vi "fitting modified.vi"(0 "fitting type":i8(ring), 5 "2D data":dbl[][](array[numeric]), 9 "force guess?":bool, 11 "intial guess value":dbl[](array[numeric])) -> (3 "number of function calls":i32 caption="function calling times", 6 "best fit":dbl[][](array[numeric]), 10 "best fit parameters":dbl[](array[numeric]), 15 "error out":errorcluster)   [LabVIEW 2015]
uses:
  <vilib>/gmath/NumericalOptimization/Nonlinear Curve Fit LM.vi
  Abort.vi
  <vilib>/gmath/NI_Gmath.lvlib
panel:
  out "Abort":bool
  in  "stop":bool
  out "Array 2":dbl[][](array[numeric])
  out "Array":i32[](array[numeric])
  out "output array":dbl[](array[numeric])
  out "size(s) 4":i32[](array[numeric])
  out "size(s) 3":i32[](array[numeric])
  out "size(s) 2":i32[](array[numeric])
  out "size(s)":i32[](array[numeric])
  out "initial value 3":dbl[](array[numeric])
  out "sub3":dbl[][](array[numeric])
  out "split 2":dbl
  out "split 1":dbl
  in  "initial value 2":dbl[](array[numeric])
  in  "initial value 1":dbl[](array[numeric])
  in  "sub2":dbl[][](array[numeric])
  in  "sub1":dbl[][](array[numeric])
  in  "yc":dbl[](array[numeric])
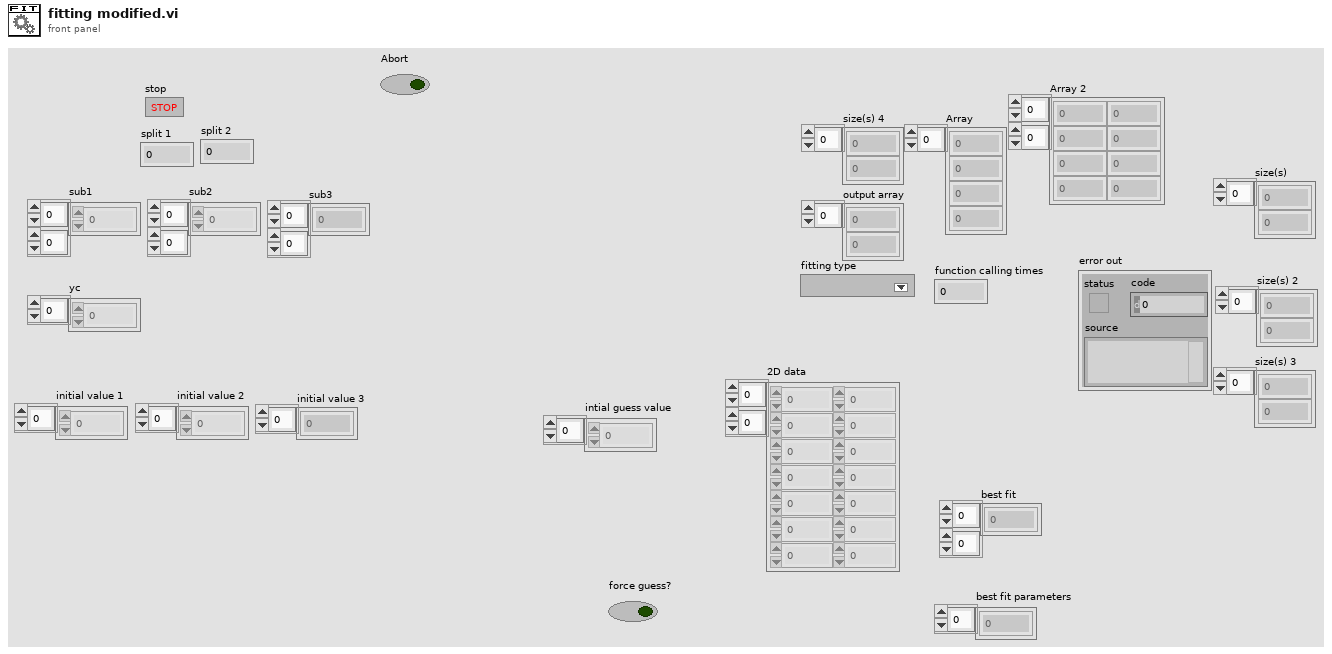
[diagram p1: front panel]
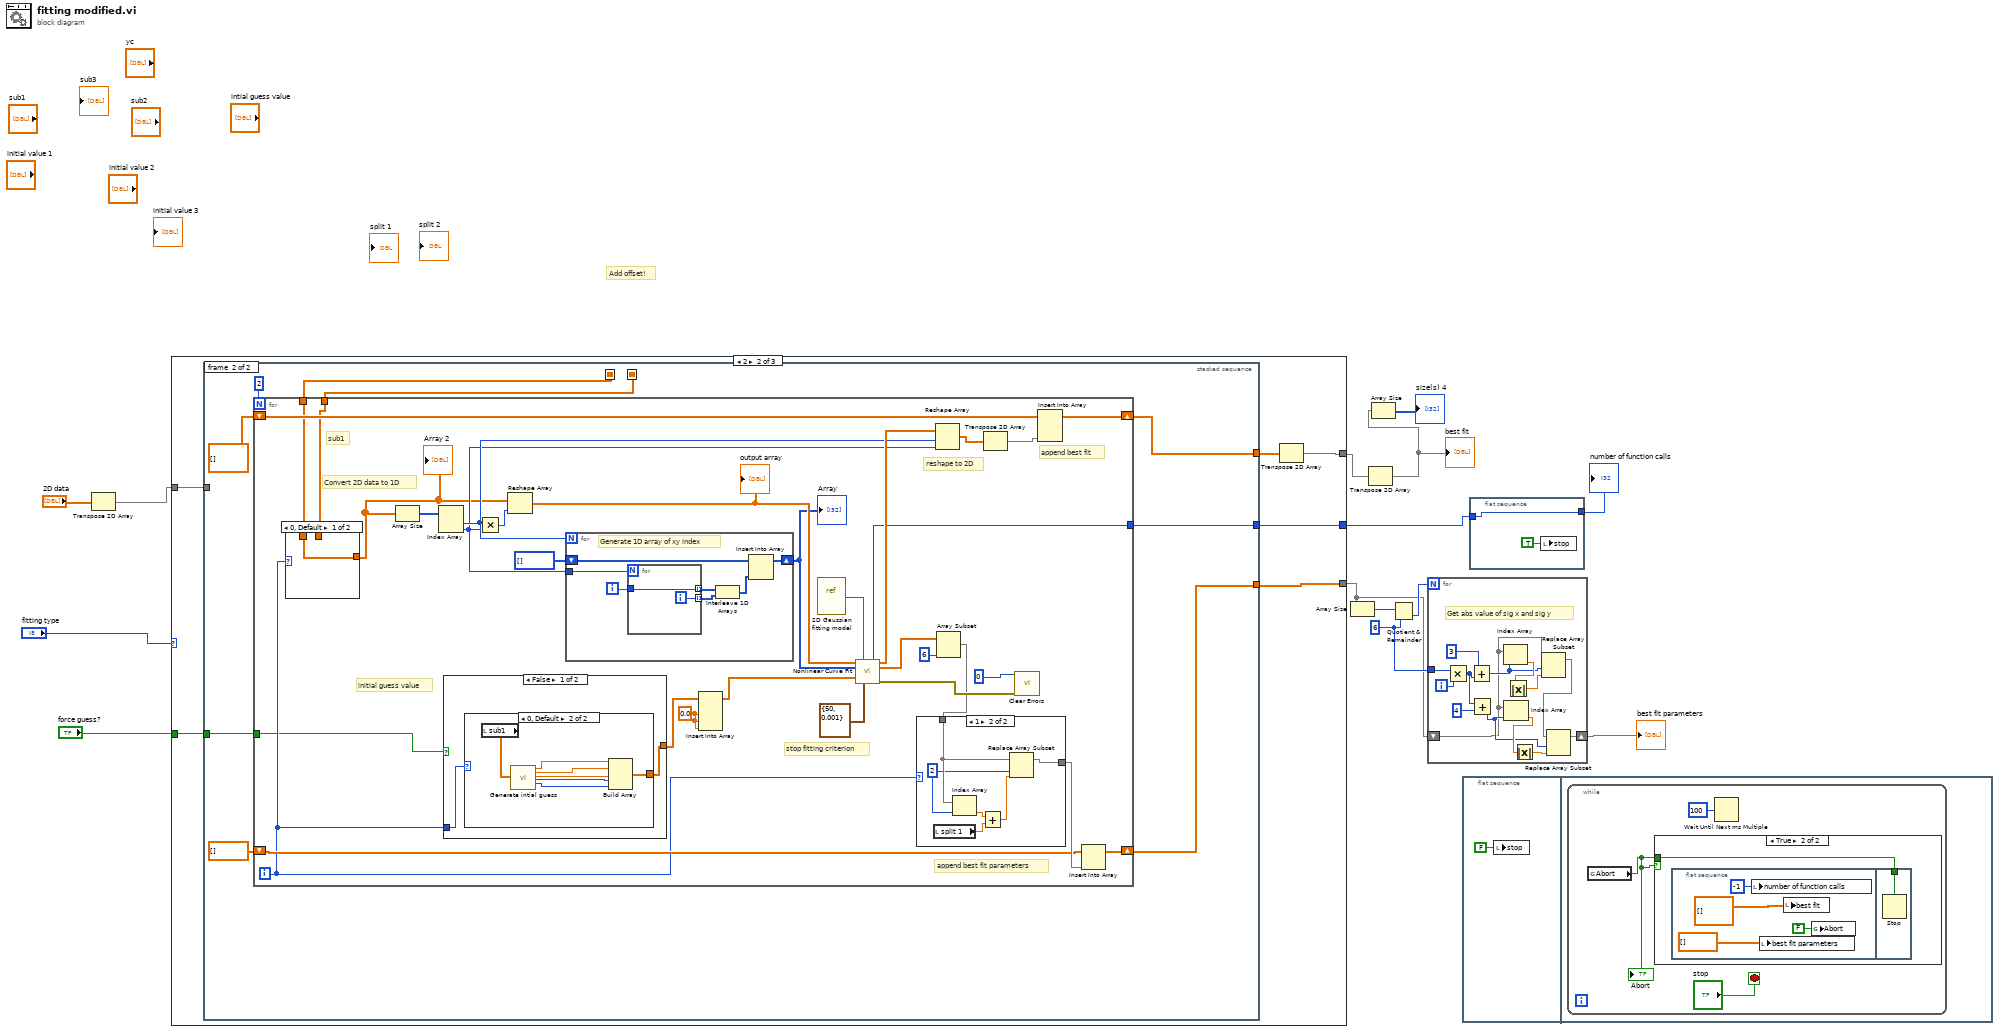
[diagram p0: block diagram]
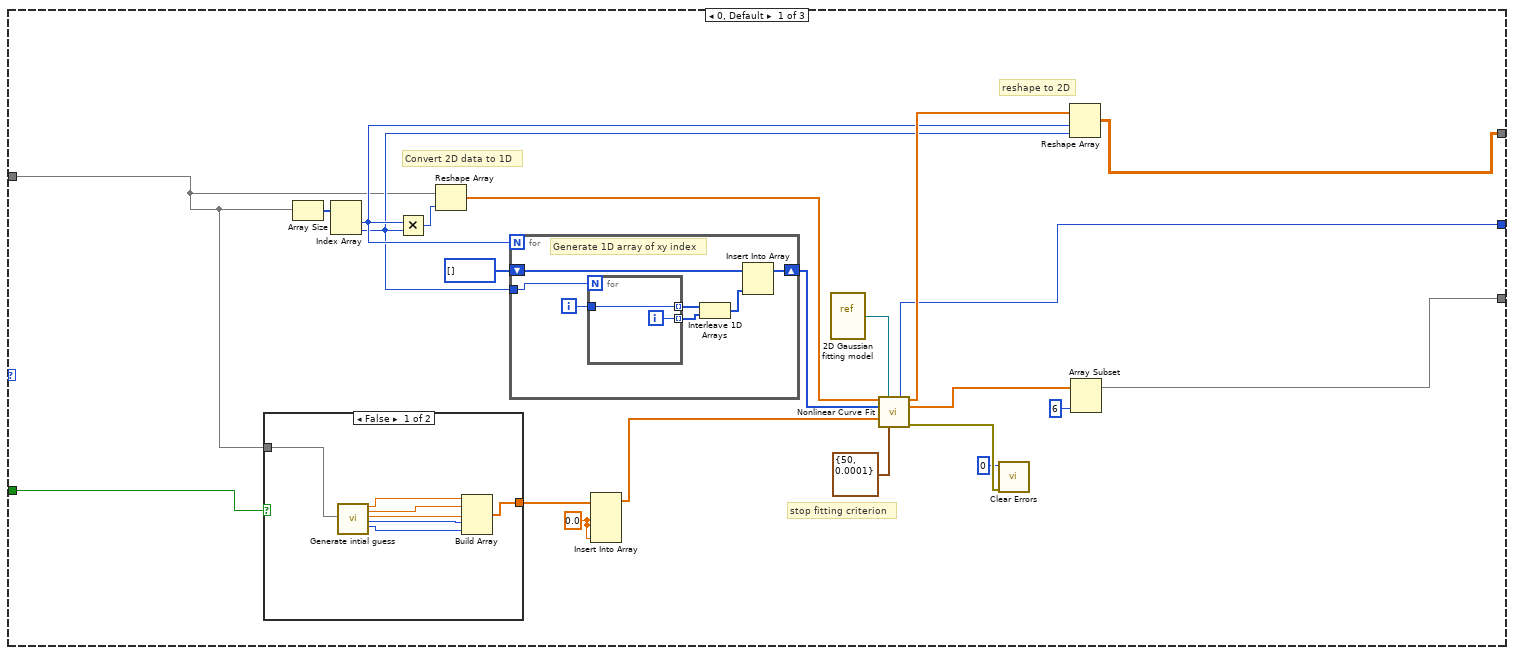
[diagram p3: hidden frame]
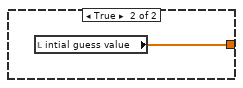
[diagram p4: hidden frame]
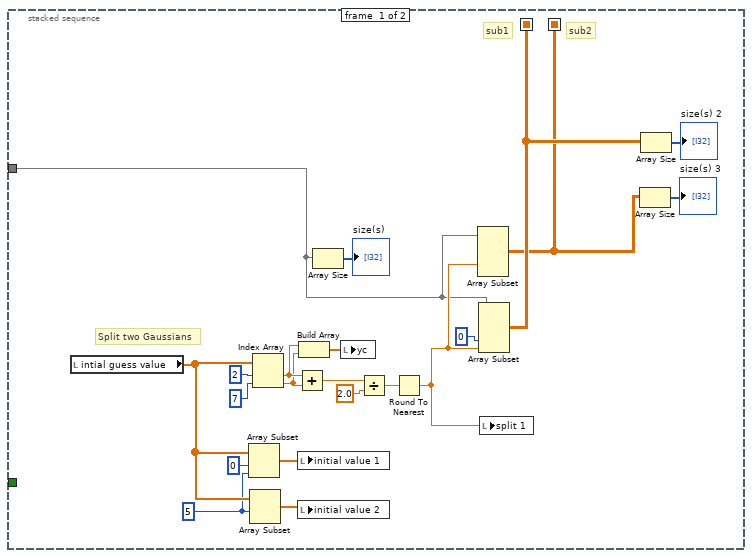
[diagram p5: hidden frame]
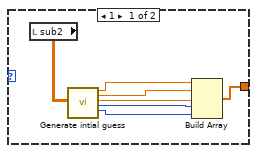
[diagram p8: hidden frame]
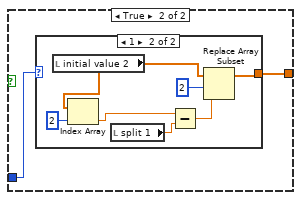
[diagram p9: hidden frame]
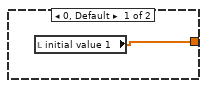
[diagram p10: hidden frame]
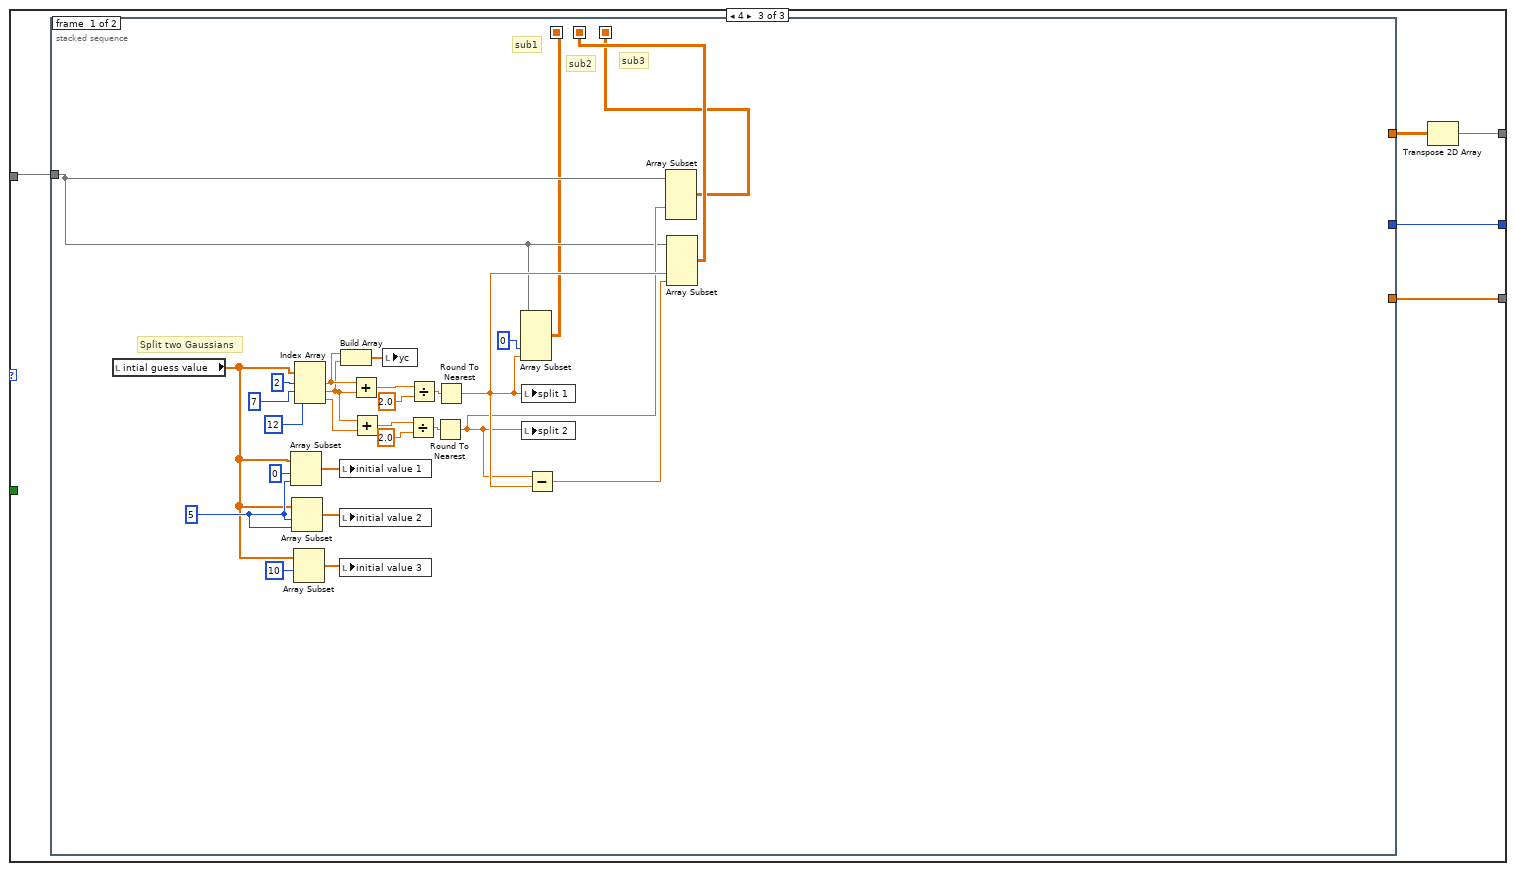
[diagram p11: hidden frame]
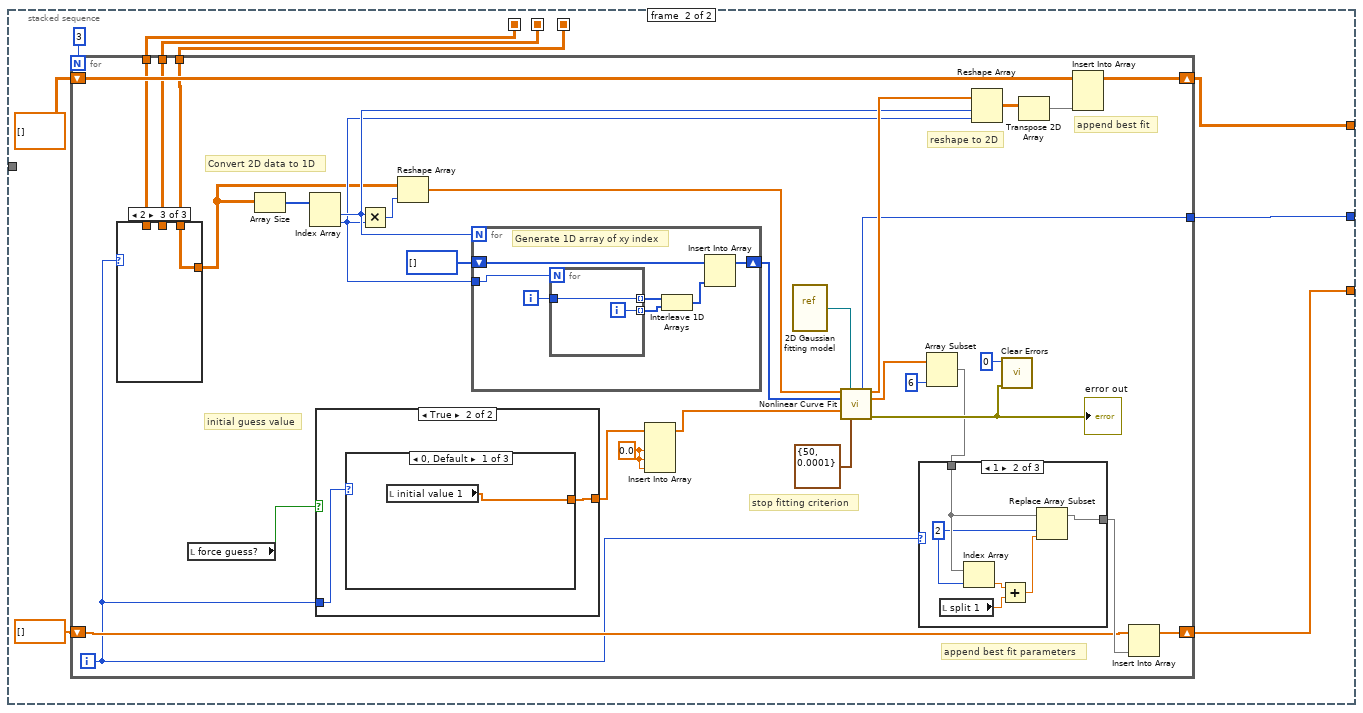
[diagram p12: hidden frame]
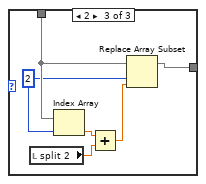
[diagram p16: hidden frame]
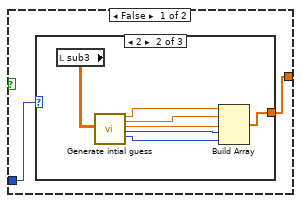
[diagram p17: hidden frame]
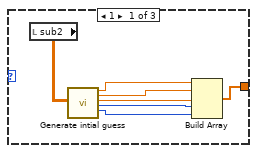
[diagram p18: hidden frame]
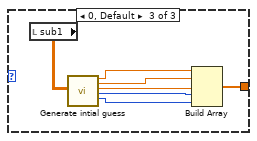
[diagram p19: hidden frame]
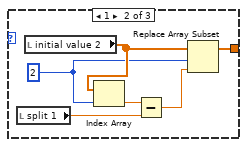
[diagram p20: hidden frame]
diagram:
  w5 = 6 ("y")
  # "Add offset!"
  n1 = Transpose 2D Array(2D array="2D data") -> (transposed array=w11:dbl[][])
  n2 = case shown="2" "fitting type" {
    tunnel: w11 -> [w24 w55 w167]
    tunnel: [w26 w54 w165] -> w9
    tunnel: [w25 w58 w169] -> w2
    tunnel: [w16 w57 w168] -> w4
    tunnel: "force guess?" -> [w23 w56 _]
    frame 0, Default {
      w20 = 0.0 ("新元素/子数组")
      # "Convert 2D data to 1D"
      # "reshape to 2D"
      # "stop fitting criterion"
      n3 = case shown="False" w23 {
        tunnel: [w47 w53] -> w22
        tunnel: w24 -> [w46 _]
        frame False {
          n4 = call "Generate intial guess.vi"("数组"=w46) -> ("peak"=w52:dbl, "xc"=w51:dbl, "yc"=w50:dbl, "sigx"=w49:i32, "sigy"=w48:i32)  [unwired: 14 in]
          n5 = Build Array(w52, w51, w50, w49, w48) -> (w47:dbl[])
        }
        frame True {
          n6 = local read "intial guess value"() -> (w53:dbl[])
        }
      }
      n7 = Array Size(array=w24) -> (size(s)=w33:i32[])
      n8 = Index Array(array=w33) -> (element #1=w29:i32, element #2=w28:i32)  [unwired: 2 in]
      n9 = Multiply(x=w29, y=w28) -> (x*y=w34:i32)
      n10 = Reshape Array(w24, w34) -> (w32:dbl[])
      n11 = for {
        N: w29 -> [_]
        shift-right: [w42] -> w27
        shift-left: i32[] [] -> [w41]
        tunnel: w28 -> [w37]
        i -> [w43]
        # "Generate 1D array of xy index"
        n12 = for {
          N: w37 -> [_]
          tunnel: [w45] -> w39 mode=indexing
          tunnel: w43 -> [w45]
          tunnel: [w44] -> w38 mode=indexing
          i -> [w44]
        }
        n13 = Interleave 1D Arrays(w39, w38) -> (w40:i32[])
        n14 = Insert Into Array(array=w41, new element=w40) -> (w42:i32[])  [unwired: 1 in]
      }
      n15 = Insert Into Array(array=w22, new element #1=w20, new element #2=w20, new element #3=w20) -> (w21:dbl[])  [unwired: 1 in]
      n16 = vi-ref "2D Gaussian fitting model.vi"() -> (w30:refnum<vi>)
      n17 = call-poly <vilib>:"Nonlinear Curve Fit.vi"("Y"=w32, "f(x,a)"=w30, "X"=w27, "initial parameters"=w21, "termination"=cluster{"max iteration":i32, "tolerance":dbl} {"max iteration"=50, "tolerance"=0.0001}) -> ("number of function calls"=w25:i32, "best nonlinear fit"=w36:dbl[], "best fit parameters"=w17:dbl[], "error out"=w19:errorcluster)  [unwired: 5 in, 2 out]
      n18 = call <vilib>:"Clear Errors.vi"("error in (no error)"=w19, "specific error code to clear (0: all)"=0) -> ()  [unwired: 4 in, 2 out]
      n19 = Reshape Array(w36, w29, w28) -> (w26:dbl[][])
      n20 = Array Subset(array=w17, length=6) -> (w16:dbl[])  [unwired: 1 in]
    }
    frame 2 {
      n21 = stacked-sequence {
        seq-local: [w64 _] -> [_ w84]
        seq-local: [w63 _] -> [_ w83]
        tunnel: [_ w81] -> w59
        tunnel: [_ w86] -> w58
        tunnel: [_ w85] -> w57
        tunnel: w56 -> [_ w82]
        tunnel: w55 -> [w60 _]
        frame #0 {
          w69 = 5 ("索引")
          # "sub2"
          # "sub1"
          # "Split two Gaussians"
          n22 = local read "intial guess value"() -> (w71:dbl[])
          n23 = Array Subset(array=w71, index=0 ("索引"), length=w69) -> (w68:dbl[])
          n24 = Array Subset(array=w71, index=w69) -> (w67:dbl[])  [unwired: 1 in]
          n25 = Index Array(array=w71, index #1=2 ("索引"), index #2=7 ("索引")) -> (element #1=w73:dbl, element #2=w72:dbl)
          n26 = Add(x=w73, y=w72) -> (x+y=w76:dbl)
          n27 = local write "initial value 1"(w68) -> ()
          n28 = local write "initial value 2"(w67) -> ()
          n29 = Build Array(w73, w72) -> (w78:dbl[])
          n30 = Array Size(array=w60) -> (size(s)=→"size(s)":i32[])
          n31 = local write "yc"(w78) -> ()
          n32 = Divide(x=w76, y=2.0) -> (x/y=w74:dbl)
          n33 = Round To Nearest(number=w74) -> (nearest integer value=w66:dbl)
          n34 = Array Subset(array=w60, index (col)=w66) -> (w63:dbl[][])  [unwired: 3 in]
          n35 = Array Subset(array=w60, index (col)=0 ("索引"), length (col)=w66) -> (w64:dbl[][])  [unwired: 2 in]
          n36 = local write "split 1"(w66) -> ()
          n37 = Array Size(array=w63) -> (size(s)=→"size(s) 3":i32[])
          n38 = Array Size(array=w64) -> (size(s)=→"size(s) 2":i32[])
        }
        frame #1 {
          n39 = for {
            N: 2 -> [_]
            shift-right: [w112] -> w81
            shift-left: dbl[][] [] -> [w111]
            shift-right: [w109] -> w85
            shift-left: dbl[] [] -> [w108]
            tunnel: [w103] -> w86
            tunnel: w84 -> [w101]
            tunnel: w83 -> [w102]
            tunnel: w82 -> [w100]
            i -> [w105]
            w95 = 0.0 ("新元素/子数组")
            # "sub1"
            # "append best fit parameters"
            # "append best fit"
            # "initial guess value"
            # "Convert 2D data to 1D"
            # "reshape to 2D"
            # "stop fitting criterion"
            n40 = case shown="0, Default" w105 {
              tunnel: [w121 w122] -> w104
              tunnel: w102 -> [_ w122]
              tunnel: w101 -> [w121 _]
              frame 0, Default {
              }
              frame 1 {
              }
            }
            "Array 2" <- w104
            n41 = Array Size(array=w104) -> (size(s)=w117:i32[])
            n42 = Index Array(array=w117) -> (element #1=w107:i32, element #2=w106:i32)  [unwired: 2 in]
            n43 = case shown="False" w100 {
              tunnel: [w140 w156] -> w99
              tunnel: w105 -> [w139 w155]
              frame False {
                n44 = case shown="0, Default" w139 {
                  tunnel: [w142 w149] -> w140
                  frame 1 {
                    n45 = local read "sub2"() -> (w141:dbl[][])
                    n46 = call "Generate intial guess.vi"("数组"=w141) -> ("peak"=w147:dbl, "xc"=w146:dbl, "yc"=w145:dbl, "sigx"=w144:i32, "sigy"=w143:i32)  [unwired: 14 in]
                    n47 = Build Array(w147, w146, w145, w144, w143) -> (w142:dbl[])
                  }
                  frame 0, Default {
                    n48 = local read "sub1"() -> (w148:dbl[][])
                    n49 = call "Generate intial guess.vi"("数组"=w148) -> ("peak"=w154:dbl, "xc"=w153:dbl, "yc"=w152:dbl, "sigx"=w151:i32, "sigy"=w150:i32)  [unwired: 14 in]
                    n50 = Build Array(w154, w153, w152, w151, w150) -> (w149:dbl[])
                  }
                }
              }
              frame True {
                n51 = case shown="1" w155 {
                  tunnel: [w157 w158] -> w156
                  frame 0, Default {
                    n52 = local read "initial value 1"() -> (w157:dbl[])
                  }
                  frame 1 {
                    n53 = local read "initial value 2"() -> (w159:dbl[])
                    n54 = Index Array(array=w159, index=2 ("索引")) -> (element=w163:dbl)
                    n55 = local read "split 1"() -> (w162:dbl)
                    n56 = Subtract(x=w163, y=w162) -> (x-y=w160:dbl)
                    n57 = Replace Array Subset(array=w159, new element=w160, index=2 ("索引")) -> (w158:dbl[])
                  }
                }
              }
            }
            n58 = Multiply(x=w107, y=w106) -> (x*y=w118:i32)
            n59 = Reshape Array(w104, w118) -> (w116:dbl[])
            "output array" <- w116
            n60 = for {
              N: w107 -> [_]
              shift-right: [w135] -> w113
              shift-left: i32[] [] -> [w134]
              tunnel: w106 -> [w130]
              i -> [w136]
              # "Generate 1D array of xy index"
              n61 = for {
                N: w130 -> [_]
                tunnel: [w138] -> w132 mode=indexing
                tunnel: w136 -> [w138]
                tunnel: [w137] -> w131 mode=indexing
                i -> [w137]
              }
              n62 = Interleave 1D Arrays(w132, w131) -> (w133:i32[])
              n63 = Insert Into Array(array=w134, new element=w133) -> (w135:i32[])  [unwired: 1 in]
            }
            "Array" <- w113
            n64 = Insert Into Array(array=w99, new element #1=w95, new element #2=w95, new element #3=w95) -> (w98:dbl[])  [unwired: 1 in]
            n65 = vi-ref "2D Gaussian fitting model.vi"() -> (w114:refnum<vi>)
            n66 = call-poly <vilib>:"Nonlinear Curve Fit.vi"("Y"=w116, "f(x,a)"=w114, "X"=w113, "initial parameters"=w98, "termination"=cluster{"max iteration":i32, "tolerance":dbl} {"max iteration"=50, "tolerance"=0.001}) -> ("number of function calls"=w103:i32, "best nonlinear fit"=w120:dbl[], "best fit parameters"=w91:dbl[], "error out"=w94:errorcluster)  [unwired: 5 in, 2 out]
            n67 = Reshape Array(w120, w107, w106) -> (w97:dbl[][])
            n68 = Array Subset(array=w91, length=6) -> (w90:dbl[])  [unwired: 1 in]
            n69 = case shown="1" w105 {
              tunnel: w90 -> [w123 w129]
              tunnel: [w123 w124] -> w110
              frame 0, Default {
              }
              frame 1 {
                w128 = 2 ("索引")
                n70 = local read "split 1"() -> (w126:dbl)
                n71 = Index Array(array=w129, index=w128) -> (element=w127:dbl)
                n72 = Add(x=w127, y=w126) -> (x+y=w125:dbl)
                n73 = Replace Array Subset(array=w129, new element=w125, index=w128) -> (w124:dbl[])
              }
            }
            n74 = Transpose 2D Array(2D array=w97) -> (transposed array=w96:dbl[][])
            n75 = call <vilib>:"Clear Errors.vi"("error in (no error)"=w94, "specific error code to clear (0: all)"=0) -> ()  [unwired: 4 in, 2 out]
            n76 = Insert Into Array(array=w111, new element=w96) -> (w112:dbl[][])  [unwired: 2 in]
            n77 = Insert Into Array(array=w108, new element=w110) -> (w109:dbl[])  [unwired: 1 in]
          }
        }
      }
      n78 = Transpose 2D Array(2D array=w59) -> (transposed array=w54:dbl[][])
    }
    frame 4 {
      n79 = stacked-sequence {
        seq-local: [w172 _] -> [_ w200]
        seq-local: [w171 _] -> [_ w199]
        seq-local: [w170 _] -> [_ w198]
        tunnel: [_ w203] -> w166
        tunnel: [_ w202] -> w169
        tunnel: [_ w201] -> w168
        tunnel: w167 -> [w173 _]
        frame #0 {
          w177 = 5 ("索引")
          # "sub3"
          # "sub2"
          # "sub1"
          # "Split two Gaussians"
          n80 = local read "intial guess value"() -> (w176:dbl[])
          n81 = Array Subset(array=w176, index=0 ("索引"), length=w177) -> (w188:dbl[])
          n82 = Array Subset(array=w176, index=w177, length=w177) -> (w187:dbl[])
          n83 = Array Subset(array=w176, index=10 ("索引")) -> (w174:dbl[])  [unwired: 1 in]
          n84 = Index Array(array=w176, index #1=2 ("索引"), index #2=7 ("索引"), index #3=12 ("索引")) -> (element #1=w190:dbl, element #2=w182:dbl, element #3=w181:dbl)
          n85 = local write "initial value 1"(w188) -> ()
          n86 = local write "initial value 2"(w187) -> ()
          n87 = local write "initial value 3"(w174) -> ()
          n88 = Build Array(w190, w182) -> (w195:dbl[])
          n89 = Add(x=w190, y=w182) -> (x+y=w193:dbl)
          n90 = Add(x=w182, y=w181) -> (x+y=w185:dbl)
          n91 = local write "yc"(w195) -> ()
          n92 = Divide(x=w185, y=2.0) -> (x/y=w183:dbl)
          n93 = Divide(x=w193, y=2.0) -> (x/y=w191:dbl)
          n94 = Round To Nearest(number=w183) -> (nearest integer value=w178:dbl)
          n95 = Round To Nearest(number=w191) -> (nearest integer value=w180:dbl)
          n96 = Array Subset(array=w173, index (col)=0 ("索引"), length (col)=w180) -> (w172:dbl[][])  [unwired: 2 in]
          n97 = local write "split 1"(w180) -> ()
          n98 = local write "split 2"(w178) -> ()
          n99 = Subtract(x=w178, y=w180) -> (x-y=w179:dbl)
          n100 = Array Subset(array=w173, index (col)=w178) -> (w170:dbl[][])  [unwired: 3 in]
          n101 = Array Subset(array=w173, index (col)=w180, length (col)=w179) -> (w171:dbl[][])  [unwired: 2 in]
        }
        frame #1 {
          n102 = for {
            N: 3 -> [_]
            shift-right: [w229] -> w203
            shift-left: dbl[][] [] -> [w228]
            shift-right: [w226] -> w201
            shift-left: dbl[] [] -> [w225]
            tunnel: [w220] -> w202
            tunnel: w200 -> [w219]
            tunnel: w199 -> [w218]
            tunnel: w198 -> [w217]
            i -> [w222]
            w210 = 0.0 ("新元素/子数组")
            # "append best fit parameters"
            # "append best fit"
            # "initial guess value"
            # "Convert 2D data to 1D"
            # "reshape to 2D"
            # "stop fitting criterion"
            n103 = case shown="2" w222 {
              tunnel: [w239 w240 w241] -> w221
              tunnel: w219 -> [w239 _ _]
              tunnel: w218 -> [_ w240 _]
              tunnel: w217 -> [_ _ w241]
              frame 0, Default {
              }
              frame 1 {
              }
              frame 2 {
              }
            }
            n104 = local read "force guess?"() -> (w236:bool)
            n105 = Array Size(array=w221) -> (size(s)=w234:i32[])
            n106 = Index Array(array=w234) -> (element #1=w224:i32, element #2=w223:i32)  [unwired: 2 in]
            n107 = case shown="True" w236 {
              tunnel: [w265 w288] -> w216
              tunnel: w222 -> [w264 w287]
              frame False {
                n108 = case shown="2" w264 {
                  tunnel: [w267 w274 w281] -> w265
                  frame 1 {
                    n109 = local read "sub2"() -> (w266:dbl[][])
                    n110 = call "Generate intial guess.vi"("数组"=w266) -> ("peak"=w272:dbl, "xc"=w271:dbl, "yc"=w270:dbl, "sigx"=w269:i32, "sigy"=w268:i32)  [unwired: 14 in]
                    n111 = Build Array(w272, w271, w270, w269, w268) -> (w267:dbl[])
                  }
                  frame 2 {
                    n112 = local read "sub3"() -> (w273:dbl[][])
                    n113 = call "Generate intial guess.vi"("数组"=w273) -> ("peak"=w279:dbl, "xc"=w278:dbl, "yc"=w277:dbl, "sigx"=w276:i32, "sigy"=w275:i32)  [unwired: 14 in]
                    n114 = Build Array(w279, w278, w277, w276, w275) -> (w274:dbl[])
                  }
                  frame 0, Default {
                    n115 = local read "sub1"() -> (w280:dbl[][])
                    n116 = call "Generate intial guess.vi"("数组"=w280) -> ("peak"=w286:dbl, "xc"=w285:dbl, "yc"=w284:dbl, "sigx"=w283:i32, "sigy"=w282:i32)  [unwired: 14 in]
                    n117 = Build Array(w286, w285, w284, w283, w282) -> (w281:dbl[])
                  }
                }
              }
              frame True {
                n118 = case shown="0, Default" w287 {
                  tunnel: [w289 w290 w296] -> w288
                  frame 0, Default {
                    n119 = local read "initial value 1"() -> (w289:dbl[])
                  }
                  frame 1 {
                    w292 = 2 ("索引")
                    n120 = local read "split 1"() -> (w294:dbl)
                    n121 = local read "initial value 2"() -> (w293:dbl[])
                    n122 = Index Array(array=w293, index=w292) -> (element=w295:dbl)
                    n123 = Subtract(x=w295, y=w294) -> (x-y=w291:dbl)
                    n124 = Replace Array Subset(array=w293, new element=w291, index=w292) -> (w290:dbl[])
                  }
                  frame 2 {
                    w298 = 2 ("索引")
                    n125 = local read "split 2"() -> (w300:dbl)
                    n126 = local read "initial value 3"() -> (w299:dbl[])
                    n127 = Index Array(array=w299, index=w298) -> (element=w301:dbl)
                    n128 = Subtract(x=w301, y=w300) -> (x-y=w297:dbl)
                    n129 = Replace Array Subset(array=w299, new element=w297, index=w298) -> (w296:dbl[])
                  }
                }
              }
            }
            n130 = Multiply(x=w224, y=w223) -> (x*y=w235:i32)
            n131 = Reshape Array(w221, w235) -> (w233:dbl[])
            n132 = for {
              N: w224 -> [_]
              shift-right: [w260] -> w230
              shift-left: i32[] [] -> [w259]
              tunnel: w223 -> [w255]
              i -> [w261]
              # "Generate 1D array of xy index"
              n133 = for {
                N: w255 -> [_]
                tunnel: [w263] -> w257 mode=indexing
                tunnel: w261 -> [w263]
                tunnel: [w262] -> w256 mode=indexing
                i -> [w262]
              }
              n134 = Interleave 1D Arrays(w257, w256) -> (w258:i32[])
              n135 = Insert Into Array(array=w259, new element=w258) -> (w260:i32[])  [unwired: 1 in]
            }
            n136 = Insert Into Array(array=w216, new element #1=w210, new element #2=w210, new element #3=w210) -> (w215:dbl[])  [unwired: 1 in]
            n137 = vi-ref "2D Gaussian fitting model.vi"() -> (w231:refnum<vi>)
            n138 = call-poly <vilib>:"Nonlinear Curve Fit.vi"("Y"=w233, "f(x,a)"=w231, "X"=w230, "initial parameters"=w215, "termination"=cluster{"max iteration":i32, "tolerance":dbl} {"max iteration"=50, "tolerance"=0.0001}) -> ("number of function calls"=w220:i32, "best nonlinear fit"=w238:dbl[], "best fit parameters"=w208:dbl[], "error out"=w214:errorcluster)  [unwired: 5 in, 2 out]
            "error out" <- w214
            n139 = Array Subset(array=w208, length=6) -> (w207:dbl[])  [unwired: 1 in]
            n140 = case shown="1" w222 {
              tunnel: w207 -> [w242 w248 w254]
              tunnel: [w242 w243 w249] -> w227
              frame 0, Default {
              }
              frame 1 {
                w247 = 2 ("索引")
                n141 = local read "split 1"() -> (w245:dbl)
                n142 = Index Array(array=w248, index=w247) -> (element=w246:dbl)
                n143 = Add(x=w246, y=w245) -> (x+y=w244:dbl)
                n144 = Replace Array Subset(array=w248, new element=w244, index=w247) -> (w243:dbl[])
              }
              frame 2 {
                w253 = 2 ("索引")
                n145 = local read "split 2"() -> (w251:dbl)
                n146 = Index Array(array=w254, index=w253) -> (element=w252:dbl)
                n147 = Add(x=w252, y=w251) -> (x+y=w250:dbl)
                n148 = Replace Array Subset(array=w254, new element=w250, index=w253) -> (w249:dbl[])
              }
            }
            n149 = Reshape Array(w238, w224, w223) -> (w212:dbl[][])
            n150 = call <vilib>:"Clear Errors.vi"("error in (no error)"=w214, "specific error code to clear (0: all)"=0) -> ()  [unwired: 4 in, 2 out]
            n151 = Transpose 2D Array(2D array=w212) -> (transposed array=w211:dbl[][])
            n152 = Insert Into Array(array=w228, new element=w211) -> (w229:dbl[][])  [unwired: 2 in]
            n153 = Insert Into Array(array=w225, new element=w227) -> (w226:dbl[])  [unwired: 1 in]
          }
        }
      }
      n154 = Transpose 2D Array(2D array=w166) -> (transposed array=w165:dbl[][])
    }
  }
  n155 = Array Size(array=w4) -> (size(s)=w7:i32)
  n156 = Transpose 2D Array(2D array=w9) -> (transposed array=w8:dbl[][])
  "best fit" <- w8
  n157 = Array Size(array=w8) -> (size(s)=→"size(s) 4":i32[])
  n158 = Quotient & Remainder(x=w7, y=w5) -> (floor(x/y)=w6:i32)  [unwired: 1 out]
  n159 = for {
    N: w6 -> [_]
    tunnel: w5 -> [w314]
    shift-right: [w303] -> w3
    shift-left: w4 -> [w302]
    i -> [w315]
    # "Get abs value of sig x and sig y"
    n160 = Multiply(x=w314, y=w315) -> (x*y=w311:i32)
    n161 = Add(x=3, y=w311) -> (x+y=w308:i32)
    n162 = Add(x=w311, y=i16 4) -> (x+y=w304:i32)
    n163 = Index Array(array=w302, index=w308) -> (element=w310:dbl)
    n164 = Index Array(array=w302, index=w304) -> (element=w306:dbl)
    n165 = Absolute Value(x=w310) -> (abs(x)=w309:dbl)
    n166 = Absolute Value(x=w306) -> (abs(x)=w305:dbl)
    n167 = Replace Array Subset(array=w302, new element=w309, index=w308) -> (w307:dbl[])
    n168 = Replace Array Subset(array=w307, new element=w305, index=w304) -> (w303:dbl[])
  }
  "best fit parameters" <- w3
  n169 = flat-sequence {
    frame #0 {
      n170 = local write "stop"(FALSE ("stop")) -> ()
    }
    frame #1 {
      n171 = while {
        stop <- "stop" stop-if-true
        n172 = global read "Abort.vi" "Abort"() -> (w317:bool)
        "Abort" <- w317
        n173 = case shown="True" w317 {
          tunnel: w317 -> [_ w320]
          frame False {
          }
          frame True {
            n174 = flat-sequence {
              tunnel: w320 -> [w325]
              frame #0 {
                n175 = local write "number of function calls"(-1 ("number of function calls")) -> ()
                n176 = local write "best fit parameters"(dbl[] [] ("Array 3")) -> ()
                n177 = local write "best fit"(dbl[][] [] ("Array 3")) -> ()
                n178 = global write "Abort.vi" "Abort"(FALSE ("Abort")) -> ()
              }
              frame #1 {
                n179 = Stop(stop? (T)=w325) -> ()
              }
            }
          }
        }
        n180 = Wait Until Next ms Multiple(millisecond multiple=u32 100) -> ()  [unwired: 1 out]
      }
    }
  }
  n181 = flat-sequence {
    tunnel: w2 -> [w327]
    tunnel: [w327] -> w1
    frame #0 {
      n182 = local write "stop"(TRUE ("stop")) -> ()
    }
  }
  "number of function calls" <- w1
